vi "__List Drag_Drop Transfer.vi"(7 "FileManager Data":T1, 8 "error in (no error)":errorcluster, 10 "Source Object":string, 11 "Source":string) -> (0 "error out":errorcluster)   [LabVIEW 2011]
doc: "This VI initiates the transfer of an object (both upload to cload and download from cloud).\nUsed to handle a transfer that results from a drag an drop operation."
uses:
  __File manager Data type.ctl
  vi.lib/National Instruments/LabVIEW Interface for Amazon S3/LV Interface for Amazon S3.lvlib
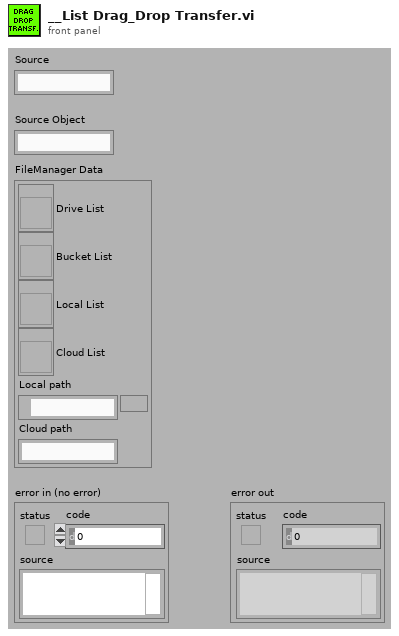
[diagram p1: front panel]
types:
  T1 = typedef "__File manager Data type.ctl" = cluster{"Drive List":refnum<vi>, "Bucket List":refnum<vi>, "Local List":refnum<vi>, "Cloud List":refnum<vi>, "Local path":path, "Cloud path":string}
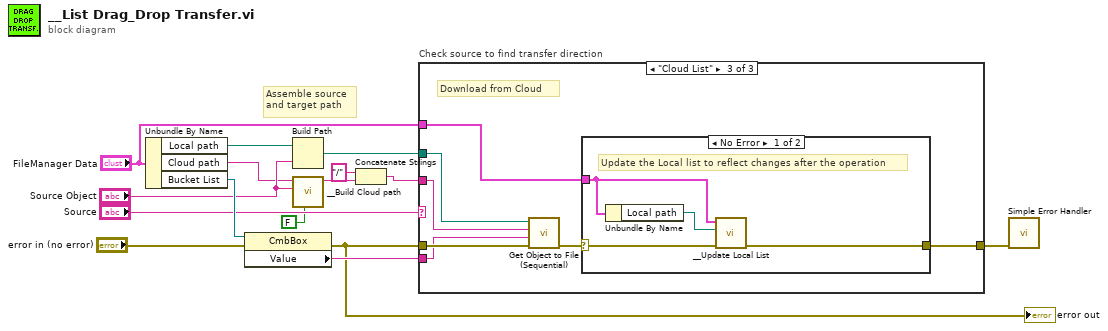
[diagram p0: block diagram]
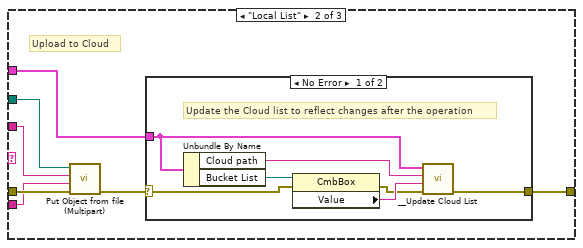
[diagram p3: hidden frame]
diagram:
  # "Assemble source\nand target path"
  n1 = Unbundle By Name("FileManager Data") -> ("Local path"=w3:path, "Cloud path"=w2:string, "Bucket List"=w14:refnum<vi>)
  n2 = property class="CmbBox"(reference=w14, error in="error in (no error)") -> (error out=w8:errorcluster, "Value"=w10:string)  [unwired: 1 out]
  "error out" <- w8
  n3 = Build Path(base path=w3, name or relative path="Source Object") -> (appended path=w11:path)
  n4 = call "__Build Cloud path.vi"("Folder?"=FALSE, "New Path element"="Source Object", "Current Cloud path"=w2) -> ("New Cloud path"=w6:string)  [unwired: 8 in]
  n5 = Concatenate Strings("/" ("string"), w6) -> (w5:string)
  n6 = case "Check source to find transfer direction" shown="\"Cloud List\"" "Source" {
    tunnel: w8 -> [w16 w23 w38]
    tunnel: [w16 w17 w32] -> w15
    tunnel: w5 -> [_ w21 w36]
    tunnel: w11 -> [_ w20 w35]
    tunnel: w10 -> [_ w22 w37]
    tunnel: "FileManager Data" -> [_ w18 w33]
    frame Default {
      # "Something is wrong! Do nothing!"
    }
    frame "Local List" {
      # "Upload to Cloud"
      n7 = call "Put Object from file (Multipart).vi"("error in (no error)"=w23, "Bucket"=w22, "Object path"=w21, "Local file path"=w20) -> ("error out"=w19:errorcluster)  [unwired: 5 in, 2 out]
      n8 = case shown="No Error" w19 {
        selector: w19 -> [w29 w31]
        tunnel: w18 -> [w25 _]
        tunnel: [w24 w31] -> w17
        frame No Error {
          # "Update the Cloud list to reflect changes after the operation"
          n9 = Unbundle By Name(w25) -> ("Cloud path"=w26:string, "Bucket List"=w30:refnum<vi>)
          n10 = property class="CmbBox"(reference=w30, error in=w29) -> (error out=w27:errorcluster, "Value"=w28:string)  [unwired: 1 out]
          n11 = call "__Update Cloud List.vi"("error in (no error)"=w27, "Bucket"=w28, "Path to list"=w26, "FileManager Ctl Refs in"=w25) -> ("error out"=w24:errorcluster)  [unwired: 6 in, 1 out]
        }
        frame Error {
        }
      }
    }
    frame "Cloud List" {
      # "Download from Cloud"
      n12 = call "Get Object to File (Sequential).vi"("error in (no error)"=w38, "Bucket"=w37, "Object Path"=w36, "File path"=w35) -> ("error out"=w34:errorcluster)  [unwired: 7 in]
      n13 = case shown="No Error" w34 {
        selector: w34 -> [w42 w43]
        tunnel: w33 -> [w40 _]
        tunnel: [w39 w43] -> w32
        frame No Error {
          # "Update the Local list to reflect changes after the operation"
          n14 = Unbundle By Name(w40) -> ("Local path"=w41:path)
          n15 = call "__Update Local List.vi"("error in (no error)"=w42, "Path to list"=w41, "FileManager Ctl Refs in"=w40) -> ("error out"=w39:errorcluster)  [unwired: 7 in, 1 out]
        }
        frame Error {
        }
      }
    }
  }
  n16 = call <vilib>:"Simple Error Handler.vi"("error in (no error)"=w15) -> ()  [unwired: 4 in, 5 out]
